vi "checkoffMissions.vi"(11 "Waypoints":refnum<queue>) -> (2 "new Mission?":bool, 3 "Waypoints out":refnum<queue>)   [LabVIEW 2013]
doc: "When there is only one waypoint left in the queue, drop the mission from the queue.\nAlso removes mission from mission queue\n\nKaitlin (4/16)"
uses:
  Classes/Waypoint/Waypoint.lvclass
  Classes/Missions/GenericMission/GenericMission.lvclass
panel:
  out "MissionArray out":refnum<class "GenericMission.lvclass">[](array[class])
  in  "MissionArray in":refnum<class "GenericMission.lvclass">[](array[class])
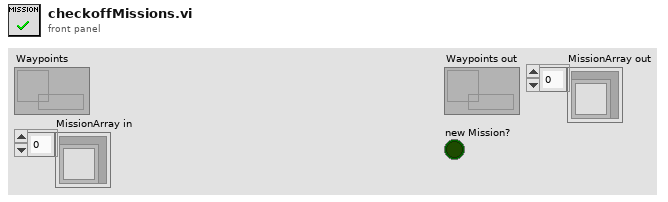
[diagram p1: front panel]
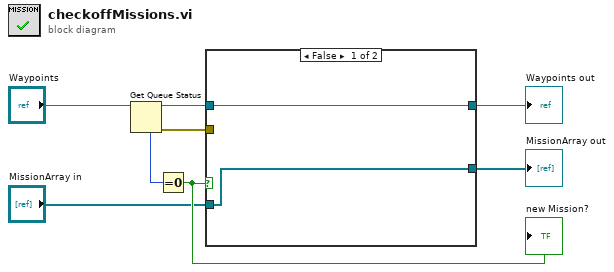
[diagram p0: block diagram]
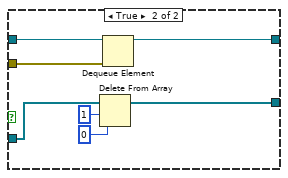
[diagram p2: hidden frame]
diagram:
  n1 = Get Queue Status(queue="Waypoints") -> (queue out=w5:refnum<queue>, error out=w4:errorcluster, # elements in queue=w7:i32)  [unwired: 2 in, 5 out]
  n2 = Equal To 0?(x=w7) -> (x = 0?=w6:bool)
  "new Mission?" <- w6
  n3 = case shown="False" w6 {
    tunnel: w5 -> [w10 w17]
    tunnel: w4 -> [_ w16]
    tunnel: [w10 w15] -> w3
    tunnel: "MissionArray in" -> [w9 w14]
    tunnel: [w9 w11] -> w1
    frame False {
    }
    frame True {
      n4 = Delete From Array(array=w14, length=1, index=0) -> (array with subset deleted=w11:refnum<class "GenericMission.lvclass">[])  [unwired: 1 out]
      n5 = Dequeue Element(queue=w17, error in (no error)=w16) -> (queue out=w15:refnum<queue>)  [unwired: 1 in, 3 out]
    }
  }
  "Waypoints out" <- w3
  "MissionArray out" <- w1
